vi "String_Array to String.vi"(6 "Seperate Blanks Items":bool, 7 "pre String In":string, 8 "Post String":string, 9 "Surround Chars":T1=enum."None;", 10 "Seperator(,)":string=",", 11 "String Array":string[](array[string])) -> (3 "String Out":string)   [LabVIEW 2015]
uses:
  TypeDefs_Utility/ENUM_String_Between tolkens.ctl
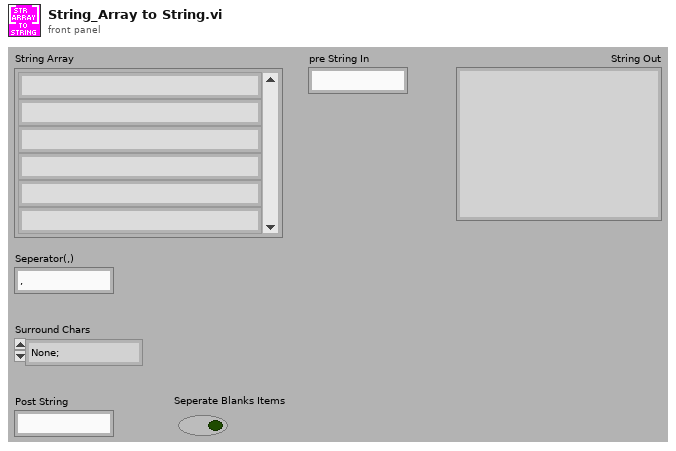
[diagram p1: front panel]
types:
  T1 = typedef "ENUM_String_Between tolkens.ctl" = enum16{"Braces;{}", "Brackets;[]", "Parens;()", "Angles;<>", "Colens;::", "Quotes;\"\"", "Backslashes;\\\\", "None;"}
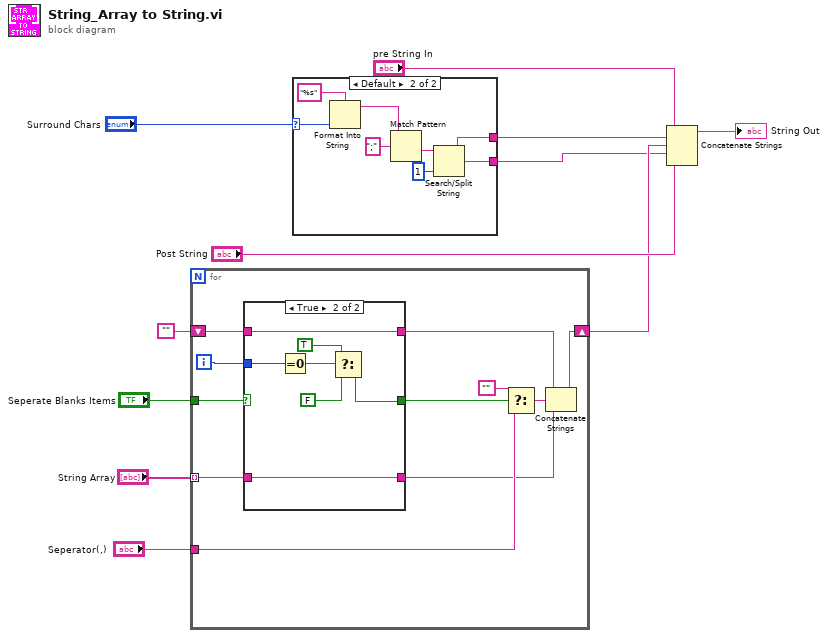
[diagram p0: block diagram]
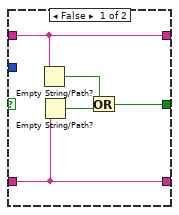
[diagram p2: hidden frame]
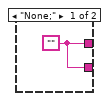
[diagram p3: hidden frame]
diagram:
  n1 = for {
    shift-right: [w22] -> w4
    shift-left: "" -> [w18]
    tunnel: "String Array" -> [w16] mode=indexing
    tunnel: "Seperator(,)" -> [w21]
    tunnel: "Seperate Blanks Items" -> [w13]
    i -> [w12]
    n2 = case shown="True" w13 {
      tunnel: w16 -> [w26 w34]
      tunnel: [w24 w29] -> w14
      tunnel: [w26 w34] -> w15
      tunnel: [w25 w33] -> w17
      tunnel: w18 -> [w25 w33]
      tunnel: w12 -> [_ w32]
      frame False {
        n3 = Empty String/Path?(string/path=w25) -> (empty?=w23:bool)
        n4 = Empty String/Path?(string/path=w26) -> (empty?=w27:bool)
        n5 = Or(x=w23, y=w27) -> (x .or. y?=w24:bool)
      }
      frame True {
        n6 = Equal To 0?(x=w32) -> (x = 0?=w31:bool)
        n7 = Select(t=TRUE, s=w31, f=FALSE) -> (s? t:f=w29:bool)
      }
    }
    n8 = Select(t="", s=w14, f=w21) -> (s? t:f=w19:string)
    n9 = Concatenate Strings(w17, w19, w15) -> (w22:string)
  }
  n10 = case shown="Default" "Surround Chars" {
    selector: "Surround Chars" -> [_ w38]
    tunnel: [w35 w40] -> w9
    tunnel: [w35 w39] -> w2
    frame "None;" {
      w35 = ""
    }
    frame Default {
      n11 = Format Into String(format string="%s", w38) -> (resulting string=w37:string)  [unwired: 2 in, 1 out]
      n12 = Match Pattern(string=w37, regular expression=";") -> (after substring=w42:string)  [unwired: 1 in, 3 out]
      n13 = Search/Split String(string=w42, offset (0)=1) -> (substring before match=w40:string, match + rest of string=w39:string)  [unwired: 1 in, 1 out]
    }
  }
  n14 = Concatenate Strings("pre String In", w9, w4, w2, "Post String") -> (→"String Out":string)
